vi "Deviation Reference Fill.vi"(8 "error in (no error)":errorcluster, 10 "Imp Parameter (F: Secondary)":bool, 11 "VISA resource name":refnum<visa-resource-name>) -> (0 "error out":errorcluster, 3 "VISA resource name out":refnum<visa-resource-name>)   [LabVIEW 2015, in "Agilent 428X Series.lvlib"]
doc: "The deviation reference fill function executes a single measurement and enters two measured values (the primary and secondary parameters) into each of the reference values for the deviation measurement."
uses:
  Agilent 428X Series.lvlib
panel:
  # "Primary\nSecondary"
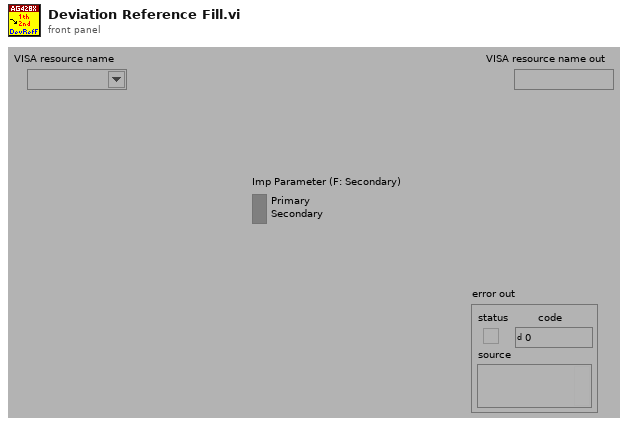
[diagram p1: front panel]
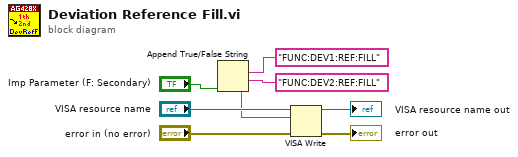
[diagram p0: block diagram]
diagram:
  n1 = Append True/False String(1:"Imp Parameter (F: Secondary)", 2:"FUNC:DEV2:REF:FILL", 3:"FUNC:DEV1:REF:FILL") -> (0:w3:string)  [unwired: 1 in]
  n2 = VISA Write(VISA resource name="VISA resource name", write buffer=w3, error in (no error)="error in (no error)") -> (VISA resource name out=→"VISA resource name out":refnum<visa-resource-name>, error out=→"error out":errorcluster)  [unwired: 1 out]
